vi "Read Sub Trees.vi"(8 "error in (no error)":errorcluster, 11 "Composite Tree in":refnum<class "Composite Tree.lvclass">) -> (0 "error out":errorcluster, 2 "Sub Trees":refnum<class "Tree.lvclass">[](array[class]), 3 "Composite Tree out":refnum<class "Composite Tree.lvclass">)   [LabVIEW 2019, in "Composite Tree.lvclass"]
uses:
  Composite Tree.lvclass
  Tree/Tree.lvclass
  Composite Tree.lvclass/Composite Tree.ctl
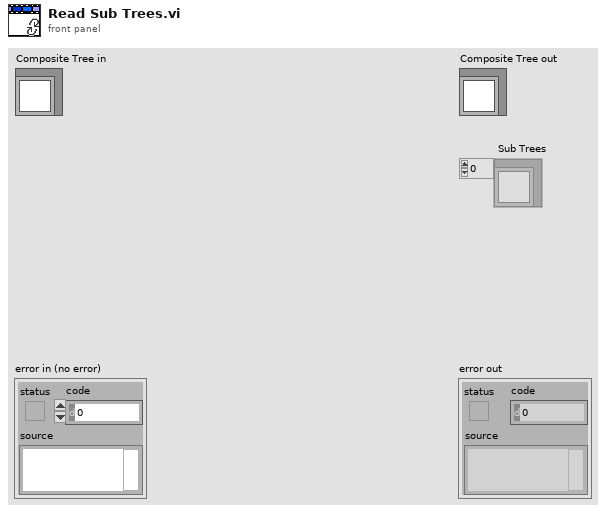
[diagram p1: front panel]
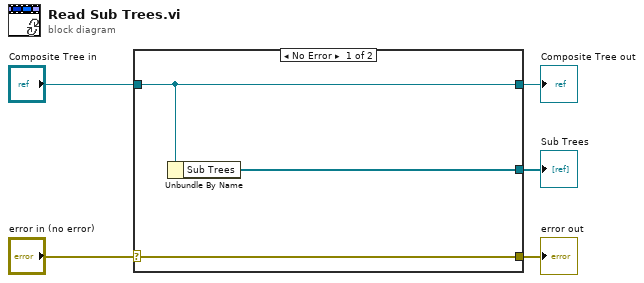
[diagram p0: block diagram]
diagram:
  n1 = case shown="No Error" "error in (no error)" {
    selector: "error in (no error)" -> [w8 w9]
    tunnel: [w8 w9] -> w4
    tunnel: [w7 w10] -> w2
    tunnel: "Composite Tree in" -> [w7 w10]
    tunnel: [w6 _] -> w1
    frame No Error {
      n2 = Unbundle By Name(w7) -> ("Sub Trees"=w6:refnum<class "Tree.lvclass">[])
    }
    frame Error {
    }
  }
  "error out" <- w4
  "Composite Tree out" <- w2
  "Sub Trees" <- w1
